vi "actions.vi"(6 "state data in":T2={"auto play?"=FALSE, "good disc?"=FALSE, "last action"=enum."start_playback", "track #"=0, "# tracks"=0, "repeat"=enum."none"}, 11 "action":T3=enum."start_playback") -> (0 "error out":errorcluster, 2 "events out":T1[](array[typedef]), 4 "state data out":T2={"auto play?"=FALSE, "good disc?"=FALSE, "last action"=enum."start_playback", "track #"=0, "# tracks"=0, "repeat"=enum."none"})   [LabVIEW 2019, in "test-state-machine.lvlib"]
uses:
  test-state-machine.lvlib
  State Data.ctl
  Action Type.ctl
  Event Type.ctl
  <vilib>/numeric/Random Number (Range) U64.vi
  <vilib>/numeric/sub_Random U32.vi
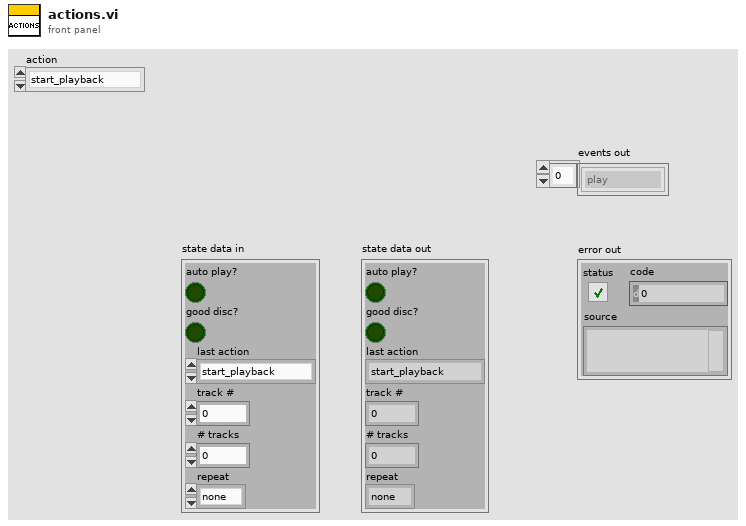
[diagram p1: front panel]
types:
  T1 = typedef "test-state-machine.lvlib/Event Type.ctl" = enum16{"play", "open_close", "stop", "cd_detected", "pause", "end_pause", "track_done", "autoplay", "error", "repeat_mode", "next", "previous"}
  T2 = typedef "test-state-machine.lvlib/State Data.ctl" = cluster{"auto play?":bool, "good disc?":bool, "last action":T3, "track #":u8, "# tracks":u8, "repeat":enum16{"none", "one", "all"}}
  T3 = typedef "test-state-machine.lvlib/Action Type.ctl" = enum16{"null action", "start_playback", "open_drawer", "close_drawer", "store_cd_info", "stop_playback", "pause_playback", "stop_and_open", "resume_playback", "next_track", "prev_track", "repeat_track", "play_first", "toggle_autoplay", "stop_safe", "toggle_repeat_mode"}
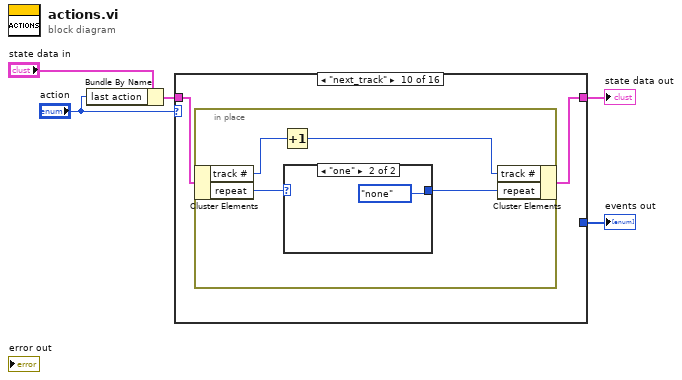
[diagram p0: block diagram]
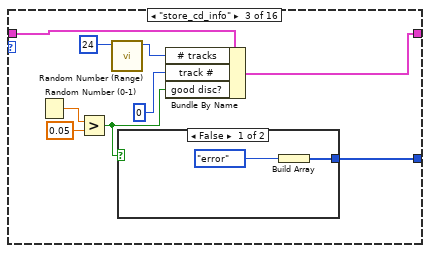
[diagram p4: hidden frame]
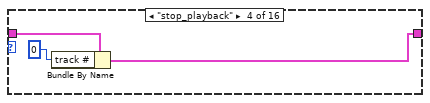
[diagram p6: hidden frame]
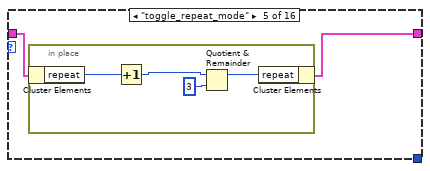
[diagram p7: hidden frame]
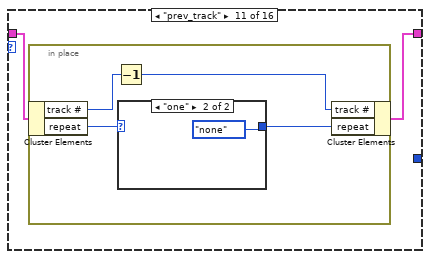
[diagram p13: hidden frame]
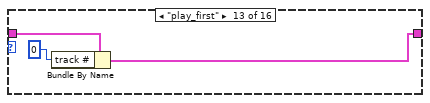
[diagram p16: hidden frame]
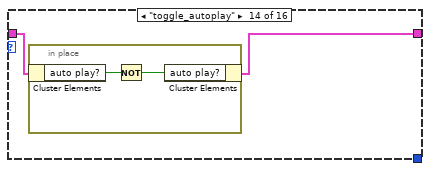
[diagram p17: hidden frame]
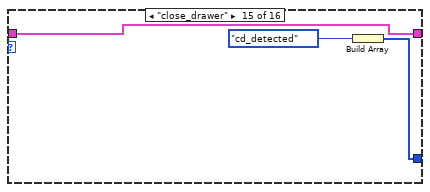
[diagram p18: hidden frame]
diagram:
  n1 = Bundle By Name(cluster="state data in", "last action"="action") -> (w3:T2)
  n2 = case shown="\"next_track\"" "action" {
    tunnel: [w6 w7 w15 w20 w22 w28 w29 w30 w31 w32 w40 w48 w50 w53 w58 w59] -> w2
    tunnel: w3 -> [w6 w7 w16 w21 w23 w28 w29 w30 w31 w33 w41 w48 w51 w52 w58 w59]
    tunnel: [_ _ w8 _ _ _ _ _ _ _ _ _ _ _ w56 _] -> w1
    frame "start_playback" {
    }
    frame "open_drawer" {
    }
    frame "store_cd_info" {
      n3 = Random Number (0-1)() -> (number: 0 to 1=w11:dbl)
      n4 = Greater?(x=w11, y=0.05) -> (0:w9:bool)
      n5 = call-poly <vilib>:"Random Number (Range).vi"("upper bound (100)"=u64 24 ("lower bound (0)")) -> ("number"=w14:u64)  [unwired: 10 in]
      n6 = case shown="False" w9 {
        tunnel: [w17 _] -> w8
        frame False {
          n7 = Build Array(Event_Type."error" ("Event Type")) -> (w17:T1[])
        }
        frame True {
        }
      }
      n8 = Bundle By Name(cluster=w16, "# tracks"=w14, "track #"=u8 0, "good disc?"=w9) -> (w15:T2)
    }
    frame "stop_playback" {
      n9 = Bundle By Name(cluster=w21, "track #"=u8 0) -> (w20:T2)
    }
    frame "toggle_repeat_mode" {
      n10 = in-place {
        n11 = in-place-cluster #1(w23) -> ("repeat"=w27:enum16{"none", "one", "all"})
        n12 = Increment(x=w27) -> (x+1=w26:enum16{"none", "one", "all"})
        n13 = Quotient & Remainder(x=w26, y=3) -> (x-y*floor(x/y)=w24:i32)  [unwired: 1 out]
        n14 = in-place-cluster #1("repeat"=w24) -> (w22:T2)
      }
    }
    frame "pause_playback" {
    }
    frame "stop_and_open" {
    }
    frame "resume_playback" {
    }
    frame "null action" {
    }
    frame "next_track" {
      n15 = in-place {
        n16 = in-place-cluster #2(w33) -> ("track #"=w37:u8, "repeat"=w35:enum16{"none", "one", "all"})
        n17 = Increment(x=w37) -> (x+1=w36:u8)
        n18 = case shown="\"one\"" w35 {
          selector: w35 -> [w38 _]
          tunnel: [w38 enum16{"none", "one", "all"}."none" ("repeat")] -> w34
          frame Default {
          }
          frame "one" {
          }
        }
        n19 = in-place-cluster #2("track #"=w36, "repeat"=w34) -> (w32:T2)
      }
    }
    frame "prev_track" {
      n20 = in-place {
        n21 = in-place-cluster #3(w41) -> ("track #"=w45:u8, "repeat"=w43:enum16{"none", "one", "all"})
        n22 = Decrement(x=w45) -> (x-1=w44:u8)
        n23 = case shown="\"one\"" w43 {
          selector: w43 -> [w46 _]
          tunnel: [w46 enum16{"none", "one", "all"}."none" ("repeat")] -> w42
          frame Default {
          }
          frame "one" {
          }
        }
        n24 = in-place-cluster #3("track #"=w44, "repeat"=w42) -> (w40:T2)
      }
    }
    frame "repeat_track" {
    }
    frame "play_first" {
      n25 = Bundle By Name(cluster=w51, "track #"=u8 0) -> (w50:T2)
    }
    frame "toggle_autoplay" {
      n26 = in-place {
        n27 = in-place-cluster #4(w52) -> ("auto play?"=w55:bool)
        n28 = Not(x=w55) -> (.not. x?=w54:bool)
        n29 = in-place-cluster #4("auto play?"=w54) -> (w53:T2)
      }
    }
    frame "close_drawer" {
      n30 = Build Array(Event_Type."cd_detected" ("Event Type")) -> (w56:T1[])
    }
    frame "stop_safe" {
    }
  }
  "state data out" <- w2
  "events out" <- w1
